vi "Get App Proj MyComp Refvi.vi"(8 "error in (no error)":errorcluster, 11 "Application in":refnum<vi>) -> (0 "error out":errorcluster, 1 "My Computer":refnum<vi>, 2 "Project Refnum":refnum<vi>, 3 "Application out":refnum<vi>)   [LabVIEW 2015, in "Generic Module Library.lvlib"]
uses:
  Generic Module Library.lvlib
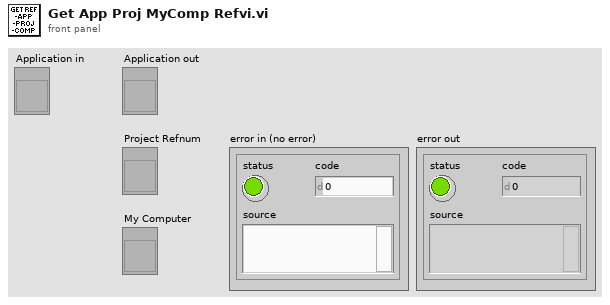
[diagram p1: front panel]
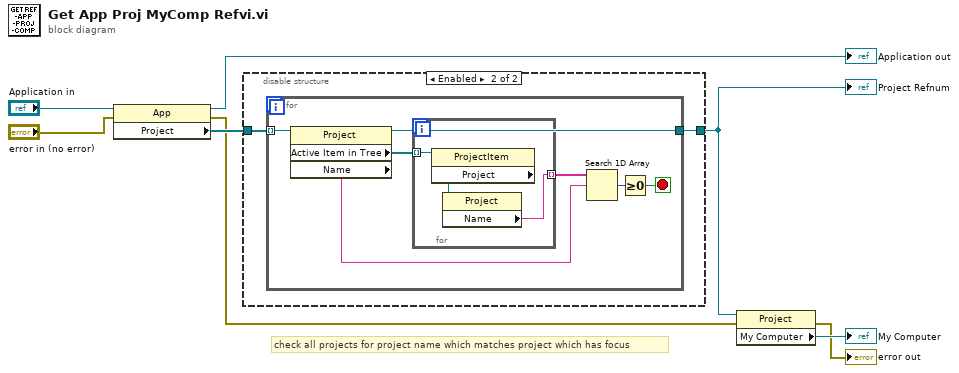
[diagram p0: block diagram]
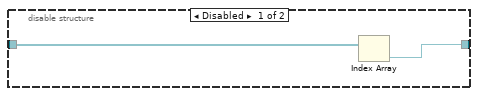
[diagram p2: hidden frame]
diagram:
  # "check all projects for project name which matches project which has focus"
  n1 = property class="App"(reference="Application in", error in="error in (no error)") -> (reference out=→"Application out":refnum<vi>, error out=w3:errorcluster, "Project"=w4:refnum<vi>[])
  n2 = disable-structure shown="Enabled" {
    disable-tunnel: [w10 w11] -> w5
    disable-tunnel: w4 -> [w9 w12]
    frame Disabled {
      n3 = Index Array(array=w9) -> (element=w10:refnum<vi>)  [unwired: 1 in]
    }
    frame Enabled {
      n4 = for {
        tunnel: w12 -> [w19] mode=indexing
        tunnel: [w16] -> w11
        stop <- w15 stop-if-true
        n5 = property class="Project"(reference=w19) -> (reference out=w16:refnum<vi>, "Active Item in Tree"=w18:refnum<vi>[], "Name"=w13:string)  [unwired: 1 in, 1 out]
        n6 = for {
          tunnel: w18 -> [w22] mode=indexing
          tunnel: [w20] -> w17 mode=indexing
          n7 = property class="ProjectItem"(reference=w22) -> ("Project"=w21:refnum<vi>)  [unwired: 1 in, 2 out]
          n8 = property class="Project"(reference=w21) -> ("Name"=w20:string)  [unwired: 1 in, 2 out]
        }
        n9 = Search 1D Array(1D array=w17, element=w13) -> (index of element=w14:i32)  [unwired: 1 in]
        n10 = Greater Or Equal To 0?(x=w14) -> (x >= 0?=w15:bool)
      }
    }
  }
  "Project Refnum" <- w5
  n11 = property class="Project"(reference=w5, error in=w3) -> (error out=→"error out":errorcluster, "My Computer"=→"My Computer":refnum<vi>)  [unwired: 1 out]
